vi "Example G-CLI (RunCaraya).vi"() -> ()   [LabVIEW 2013]
uses:
  <vilib>/Utility/sysdir.llb/System Directory Type.ctl
panel:
  in  "Exit when done?":bool
  out "return code":i32
  out "standard output":string
  in  "LabVIEW Version":u16=2019
  out "Command Line string":string
  in  "Output file":path
  out "error out":errorcluster
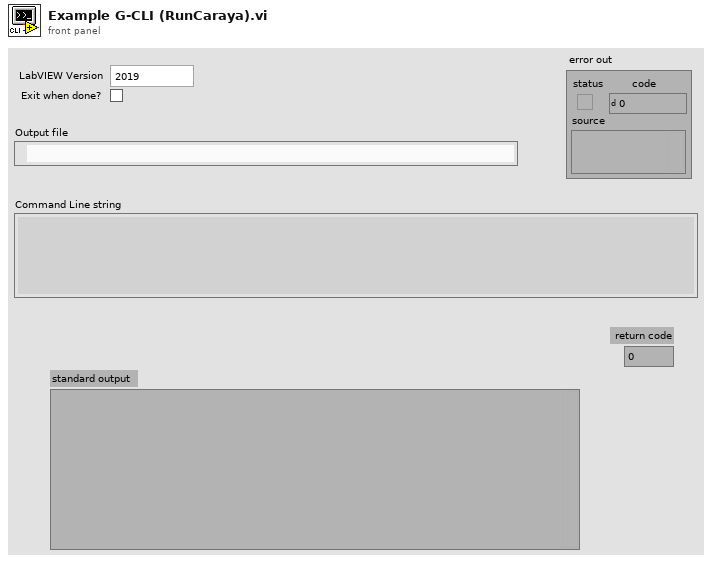
[diagram p1: front panel]
types:
  T1 = typedef "System Directory Type.ctl" = i32
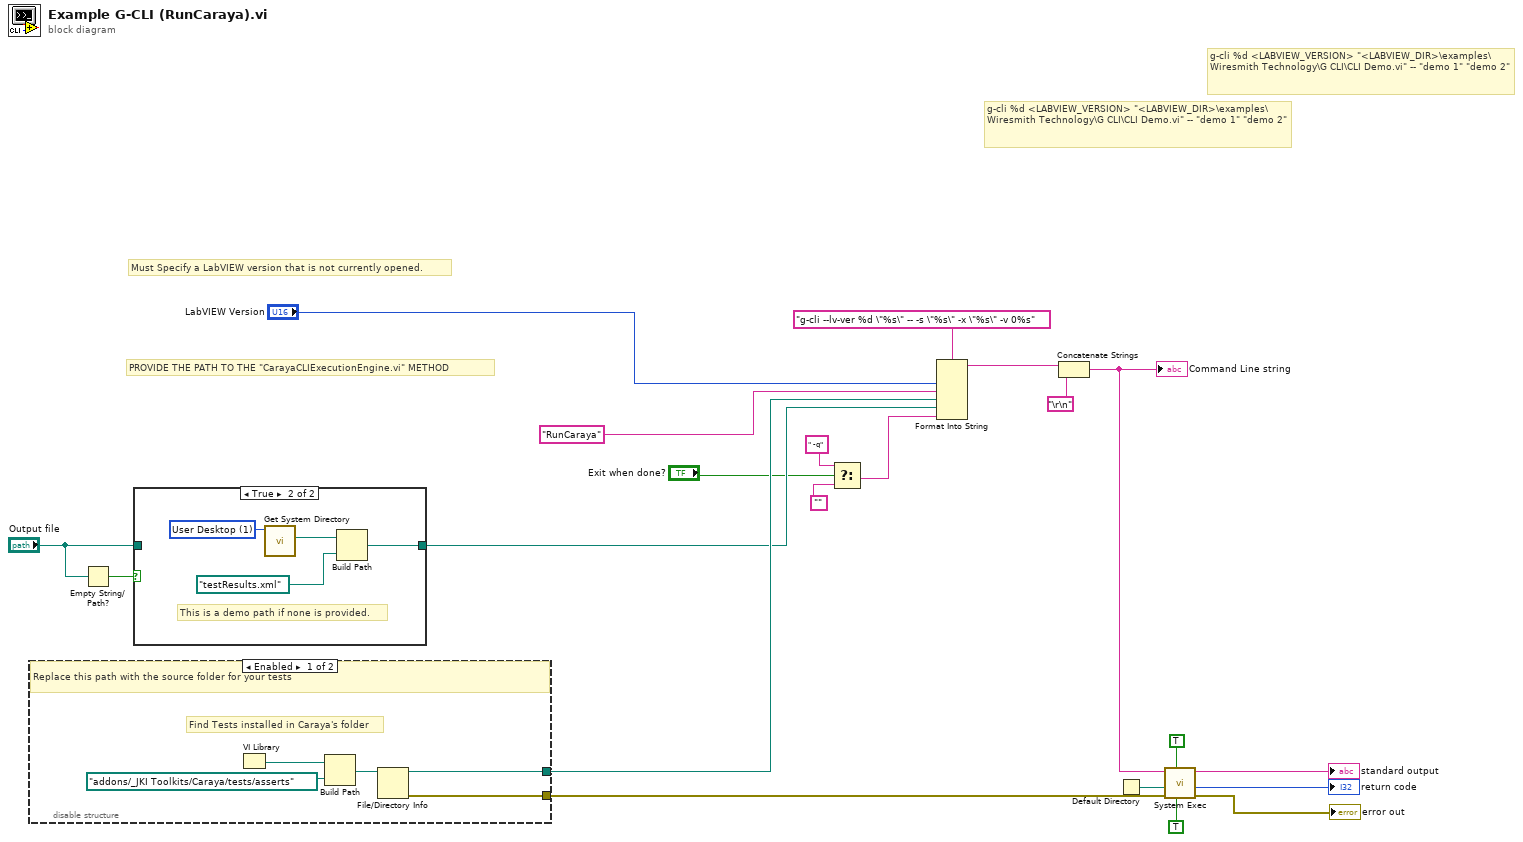
[diagram p0: block diagram]
diagram:
  # "PROVIDE THE PATH TO THE \"CarayaCLIExecutionEngine.vi\" METHOD"
  # "g-cli %d <LABVIEW_VERSION> \"<LABVIEW_DIR>\\examples\\Wiresmith Technology\\G CLI\\CLI Demo.vi\" -- \"demo 1\" \"demo 2\""
  # "g-cli %d <LABVIEW_VERSION> \"<LABVIEW_DIR>\\examples\\Wiresmith Technology\\G CLI\\CLI Demo.vi\" -- \"demo 1\" \"demo 2\""
  # "Must Specify a LabVIEW version that is not currently opened."
  n1 = disable-structure shown="Enabled" {
    disable-tunnel: [w26 _] -> w10
    disable-tunnel: [w22 _] -> w6
    frame Enabled {
      # "Find Tests installed in Caraya's folder"
      # "Replace this path with the source folder for your tests"
      n2 = VI Library() -> (path=w25:path)
      n3 = Build Path(base path=w25, name or relative path=path "addons/_JKI Toolkits/Caraya/tests/asserts") -> (appended path=w23:path)
      n4 = File/Directory Info(path=w23) -> (path out=w26:path, error out=w22:errorcluster)  [unwired: 1 in, 5 out]
    }
    frame Disabled {
    }
  }
  n5 = Empty String/Path?(string/path="Output file") -> (empty?=w13:bool)
  n6 = case shown="True" w13 {
    tunnel: [w27 w29] -> w7
    tunnel: "Output file" -> [w27 _]
    frame False {
    }
    frame True {
      w31 = T1 1 items=["User Home"=0, "User Desktop"=1, "User Documents"=2, "User Application Data"=3, "User Preferences"=4, "User Temporary"=5, "Public Documents"=6, "Public Application Data"=7, "Public Preferences"=8, "Public Cache"=13, "System Core Libraries"=9, "System Installed Libraries"=10, "Application Files"=11, "Boot Volume Root"=12] ("system directory type")
      # "This is a demo path if none is provided."
      n7 = call <vilib>:"Get System Directory.vi"("system directory type"=w31) -> ("system directory"=w28:path)  [unwired: 10 in]
      n8 = Build Path(base path=w28, name or relative path=path "testResults.xml") -> (appended path=w29:path)
    }
  }
  n9 = Select(t=" -q" ("format string"), s="Exit when done?", f="") -> (s? t:f=w2:string)
  n10 = Format Into String(format string="g-cli --lv-ver %d \"%s\" -- -s \"%s\" -x \"%s\" -v 0%s", "LabVIEW Version", "RunCaraya" ("format string"), w10, w7, w2) -> (resulting string=w15:string)  [unwired: 2 in, 1 out]
  n11 = Concatenate Strings(w15, "\r\n") -> (w17:string)
  "Command Line string" <- w17
  n12 = Default Directory() -> (w14:path)
  n13 = call <vilib>:"System Exec.vi"("run minimized? (F)"=TRUE, "wait until completion? (T)"=TRUE, "error in (no error)"=w6, "working directory"=w14, "command line"=w17) -> ("error out"=→"error out":errorcluster, "return code"=→"return code":i32, "standard output"=→"standard output":string)  [unwired: 3 in, 1 out]
